vi "CreateTracker.vi"(1 "height":u32=256, 2 "width":u32=256) -> (0 "return type":u64)   [LabVIEW 2011]
uses:
  TrackerDLL.vi
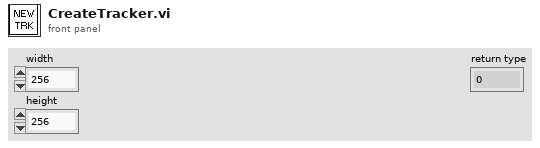
[diagram p1: front panel]
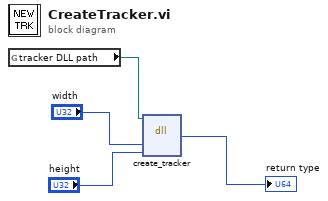
[diagram p0: block diagram]
diagram:
  n1 = global read "TrackerDLL.vi" "tracker DLL path"() -> (w1:path)
  n2 = dll-call lib="D:/jcnossen1/cudaqi-tracker/Debug/cputrack.dll" fn="create_tracker"(path in=w1, "width"="width", "height"="height") -> ("return type"=→"return type":u64)  [unwired: 4 in, 2 out]
